vi "main.vi"() -> ()   [LabVIEW 2010]
uses:
  CPES_Control.ctl
  MainStateQueueType.ctl
  MainStates.ctl
  <vilib>/Utility/miscctls.llb/LVBoundsTypeDef.ctl
  MainGlobalConstants.vi
panel:
  in  "OK Button 8":bool
  in  "OK Button 7":bool
  in  "OK Button 6":bool
  in  "OK Button 5":bool
  in  "医学3D成像":bool
  in  "模糊控制实验":bool
  in  "工业转子平台":bool
  in  "工业过程测量":bool
  in  "精准农业":bool
  in  "CPES":T1
  # "智能测试与传感网络研究室综合平台"
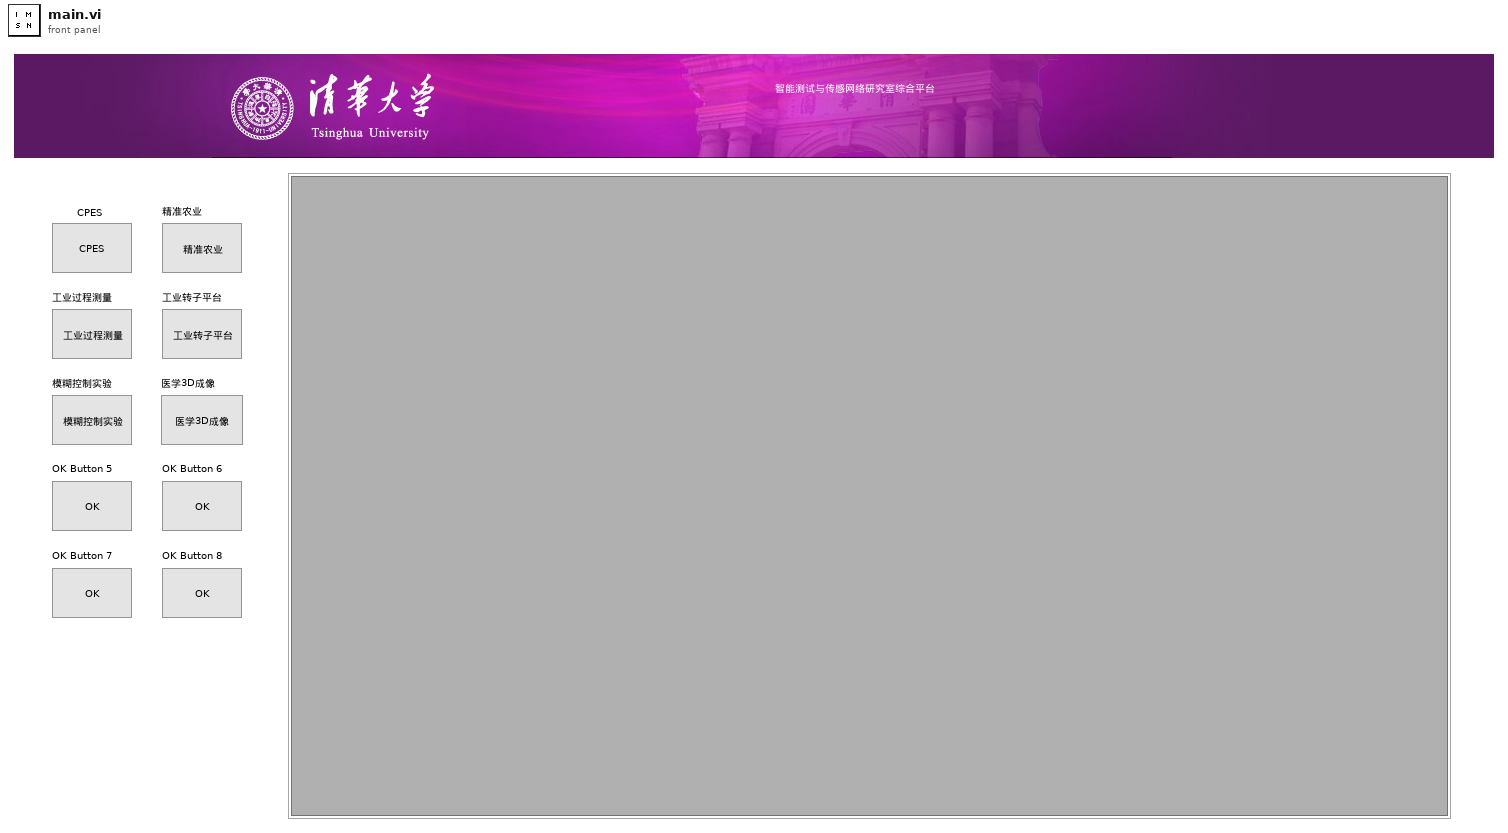
[diagram p1: front panel]
types:
  T1 = typedef "CPES_Control.ctl" = bool
  T2 = typedef "MainStateQueueType.ctl" = cluster{"Data":variant, "MainState":T3}
  T3 = typedef "MainStates.ctl" = enum16{"initMain", "insertSubVI", "startSubVI", "stopSubVI", "Exit", "ERROR", "idle"}
  T4 = typedef "LVBoundsTypeDef.ctl" = cluster{"Width":u32, "Height":u32}
  T5 = enum32{"Bad", "Idle", "Run top level", "Running"}
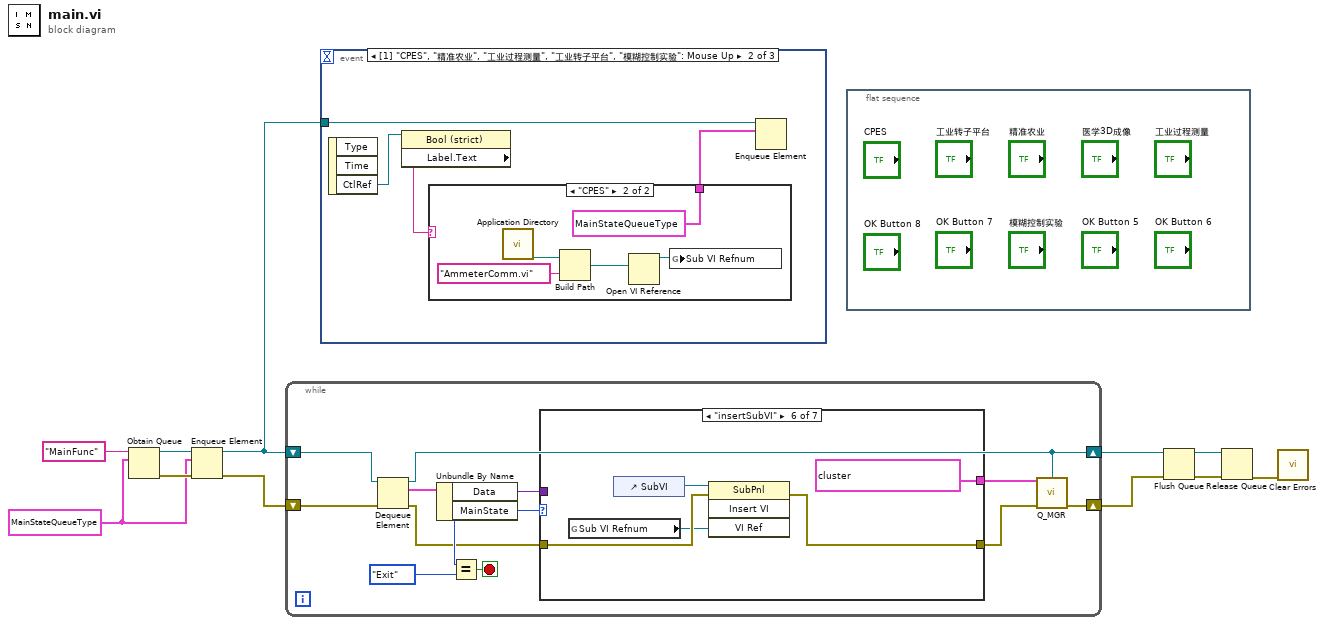
[diagram p0: block diagram]
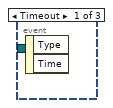
[diagram p2: hidden frame]
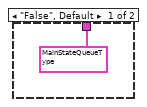
[diagram p3: hidden frame]
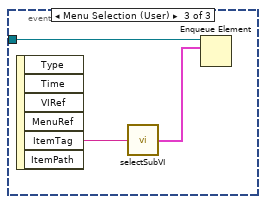
[diagram p4: hidden frame]
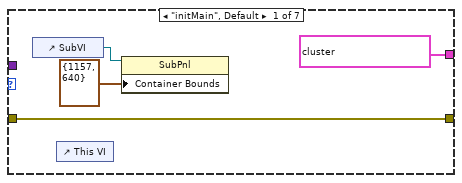
[diagram p5: hidden frame]
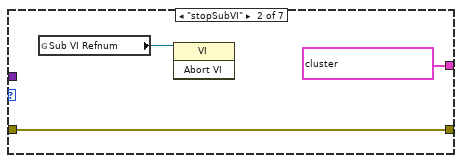
[diagram p6: hidden frame]
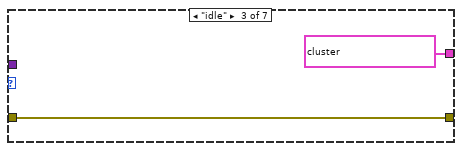
[diagram p7: hidden frame]
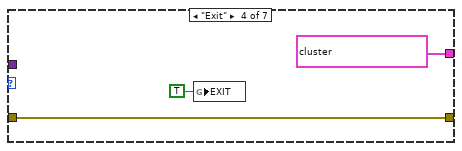
[diagram p8: hidden frame]
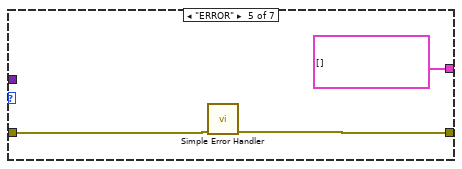
[diagram p9: hidden frame]
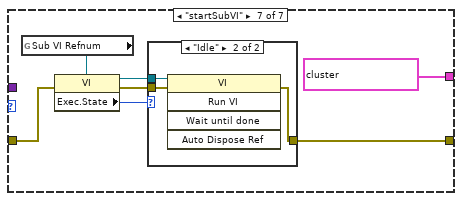
[diagram p10: hidden frame]
diagram:
  w6 = T2 {"Data"=variant, "MainState"=enum."initMain"} ("MainStateQueue")
  n1 = Obtain Queue(name (unnamed)="MainFunc", element data type=w6) -> (queue out=w10:refnum<queue>, error out=w11:errorcluster)  [unwired: 3 in, 1 out]
  n2 = Enqueue Element(queue=w10, element=w6, error in (no error)=w11) -> (queue out=w8:refnum<queue>, error out=w7:errorcluster)  [unwired: 1 in, 1 out]
  n3 = while {
    shift-right: [w13] -> w5
    shift-left: w8 -> [w22]
    shift-right: [w14] -> w2
    shift-left: w7 -> [w20]
    stop <- w21 stop-if-true
    n4 = Dequeue Element(queue=w22, error in (no error)=w20) -> (queue out=w13:refnum<queue>, element=w23:T2, error out=w17:errorcluster)  [unwired: 1 in, 1 out]
    n5 = Unbundle By Name(w23) -> ("Data"=w16:variant, "MainState"=w18:T3)
    n6 = Equal?(x=w18, y=MainStates."Exit" ("Ring")) -> (x = y?=w21:bool)
    n7 = case shown="\"insertSubVI\"" w18 {
      tunnel: w17 -> [w27 w30 w32 w33 w38 w43 w47]
      tunnel: [w27 w30 w32 w33 w37 w42 w50] -> w15
      tunnel: w16 -> [_ _ _ _ _ _ _]
      tunnel: [cluster{"Data":variant, "MainState":T3}[] [{"Data"=variant, "MainState"=enum."idle"}] ("QSTATES") cluster{"Data":variant, "MainState":T3}[] [{"Data"=variant, "MainState"=enum."idle"}] ("QSTATES") cluster{"Data":variant, "MainState":T3}[] [{"Data"=variant, "MainState"=enum."idle"}] ("QSTATES") cluster{"Data":variant, "MainState":T3}[] [{"Data"=variant, "MainState"=enum."Exit"}] ("QSTATES") cluster{"Data":variant, "MainState":T3}[] [] ("QSTATES") cluster{"Data":variant, "MainState":T3}[] [{"Data"=variant, "MainState"=enum."startSubVI"}] ("QSTATES") cluster{"Data":variant, "MainState":T3}[] [{"Data"=variant, "MainState"=enum."idle"}] ("QSTATES")] -> w12
      frame "initMain", Default {
        n8 = control-ref of="SubVI"() -> (w25:refnum<vi>)
        n9 = control-ref of="This VI"() -> ()  [unwired: 1 out]
        n10 = property class="SubPnl"(reference=w25, "Container Bounds"=T4 {"Width"=1157, "Height"=640}) -> ()  [unwired: 1 in, 2 out]
      }
      frame "stopSubVI" {
        n11 = global read "MainGlobalConstants.vi" "Sub VI Refnum"() -> (w29:refnum<vi>)
        n12 = invoke class="VI" method="Abort VI"(reference=w29) -> ()  [unwired: 2 in, 3 out]
      }
      frame "idle" {
      }
      frame "Exit" {
        n13 = global write "MainGlobalConstants.vi" "EXIT"(TRUE ("EXIT")) -> ()
      }
      frame "ERROR" {
        n14 = call <vilib>:"Simple Error Handler.vi"("error in (no error)"=w38) -> ("error out"=w37:errorcluster)  [unwired: 4 in, 4 out]
      }
      frame "insertSubVI" {
        n15 = global read "MainGlobalConstants.vi" "Sub VI Refnum"() -> (w39:refnum<vi>)
        n16 = control-ref of="SubVI"() -> (w40:refnum<vi>)
        n17 = invoke class="SubPnl" method="Insert VI"(reference=w40, error in=w43, "VI Ref"=w39) -> (error out=w42:errorcluster)  [unwired: 1 in, 3 out]
      }
      frame "startSubVI" {
        n18 = global read "MainGlobalConstants.vi" "Sub VI Refnum"() -> (w49:refnum<vi>)
        n19 = property class="VI"(reference=w49, error in=w47) -> (reference out=w48:refnum<vi>, error out=w46:errorcluster, "Exec.State"=w45:T5)
        n20 = case shown="\"Idle\"" w45 {
          tunnel: [w51 w52] -> w50
          tunnel: w48 -> [_ w54]
          tunnel: w46 -> [w51 w53]
          frame "Bad", Default {
          }
          frame "Idle" {
            n21 = invoke class="VI" method="Run VI"(reference=w54, error in=w53) -> (error out=w52:errorcluster)  [unwired: 3 in, 4 out]
          }
        }
      }
    }
    n22 = call "Q_MGR.vi"("QSTATES"=w12, "QRef"=w13, "Error IN"=w15) -> ("Error OUT"=w14:errorcluster)  [unwired: 12 in]
  }
  n23 = event shown="[1] \"CPES\", \"精准农业\", \"工业过程测量\", \"工业转子平台\", \"模糊控制实验\": Mouse Up" {
    selector: _ -> [_ _ _]
    dyn-events: _ -> [_ _ _]
    timeout: _ -> [_ _ _]
    tunnel: w8 -> [_ w58 w66]
    event Timeout {
      n24 = event-data() -> ()  [unwired: 1 in, 2 out]
    }
    event "精准农业", "工业过程测量", "工业转子平台", "模糊控制实验": Mouse Up {
      n25 = event-data() -> ("CtlRef"=w57:refnum<vi>)  [unwired: 1 in, 2 out]
      n26 = property class="Bool (strict)"(reference=w57) -> ("Label.Text"=w56:string)  [unwired: 1 in, 2 out]
      n27 = case shown="\"CPES\"" w56 {
        tunnel: [T2 {"Data"=variant, "MainState"=enum."idle"} ("MainStateQueue") T2 {"Data"=variant, "MainState"=enum."insertSubVI"} ("MainStateQueue")] -> w55
        frame "False", Default {
        }
        frame "CPES" {
          n28 = call <vilib>:"Application Directory.vi"() -> ("Application Directory"=w64:path)
          n29 = Build Path(base path=w64, name or relative path="AmmeterComm.vi") -> (appended path=w62:path)
          n30 = Open VI Reference(vi path=w62) -> (vi reference=w60:refnum<vi>)  [unwired: 5 in, 1 out]
          n31 = global write "MainGlobalConstants.vi" "Sub VI Refnum"(w60) -> ()
        }
      }
      n32 = Enqueue Element(queue=w58, element=w55) -> ()  [unwired: 2 in, 3 out]
    }
    event Menu Selection (User) {
      n33 = event-data() -> ("ItemTag"=w67:string)  [unwired: 1 in, 5 out]
      n34 = call "selectSubVI.vi"("ItemTag"=w67) -> ("MainStateQueue"=w65:T2)
      n35 = Enqueue Element(queue=w66, element=w65) -> ()  [unwired: 2 in, 3 out]
    }
  }
  n36 = flat-sequence {
    frame #0 {
    }
  }
  n37 = Flush Queue(queue=w5, error in (no error)=w2) -> (queue out=w3:refnum<queue>, error out=w1:errorcluster)  [unwired: 1 out]
  n38 = Release Queue(queue=w3, error in (no error)=w1) -> (error out=w4:errorcluster)  [unwired: 1 in, 2 out]
  n39 = call <vilib>:"Clear Errors.vi"("error in (no error)"=w4) -> ()  [unwired: 6 in, 1 out]
